vi "FileFunctions.AddDateToFile.vi"   [LabVIEW 2016]
types:
  T1 = enum16{"open", "replace", "create", "open or create", "replace or create", "replace or create with confirmation"}
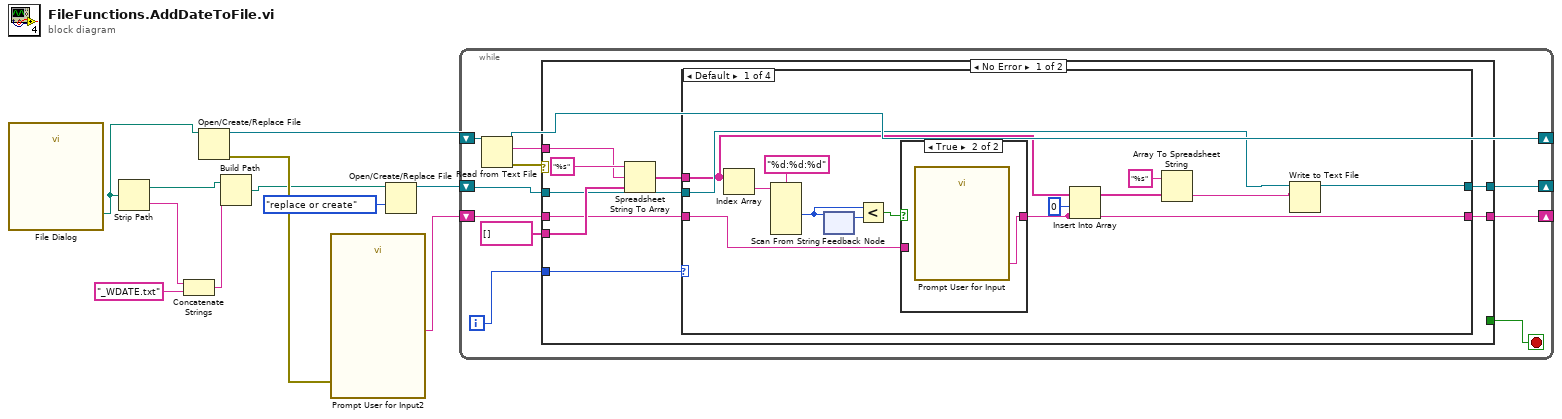
[diagram p0: block diagram]
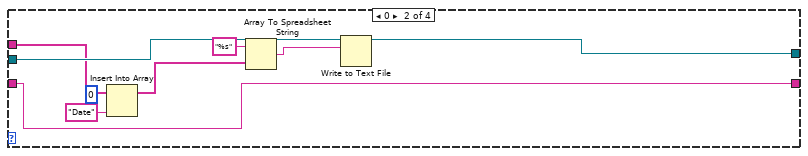
[diagram p3: hidden frame]
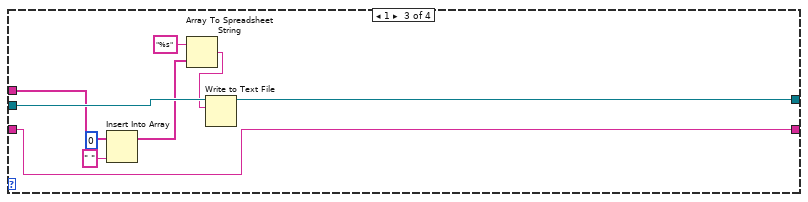
[diagram p4: hidden frame]
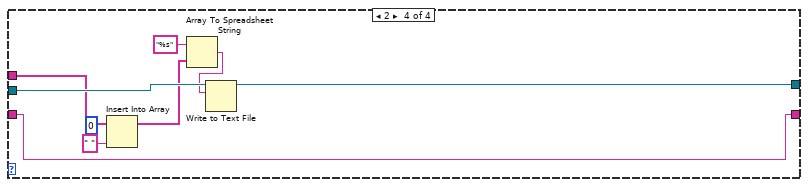
[diagram p5: hidden frame]
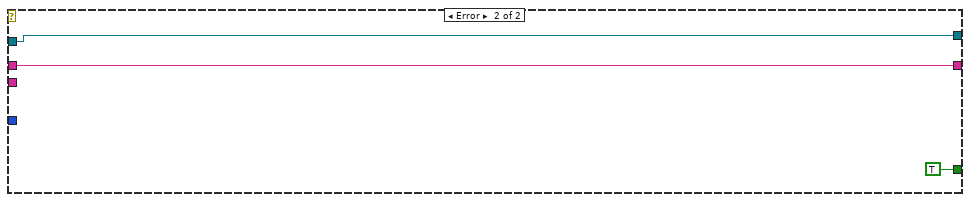
[diagram p6: hidden frame]
diagram:
  n1 = call "File Dialog"() -> ("selected path"=w6:path)  [unwired: 12 in, 3 out]
  n2 = Strip Path(path=w6) -> (stripped path=w5:path, name=w4:string)
  n3 = Concatenate Strings(w4, "_WDATE.txt" ("string")) -> (w3:string)
  n4 = Open/Create/Replace File(file path (use dialog)=w6) -> (refnum out=w7:refnum<file>, error out=w9:errorcluster)  [unwired: 5 in, 1 out]
  n5 = Build Path(base path=w5, name or relative path=w3) -> (appended path=w1:path)
  n6 = call "Prompt User for Input2"("error in (no error)"=w9) -> ("Date"=w8:string)  [unwired: 16 in, 2 out]
  n7 = Open/Create/Replace File(file path (use dialog)=w1, operation (0:open)=T1."replace or create") -> (refnum out=w11:refnum<file>)  [unwired: 4 in, 2 out]
  n8 = while {
    shift-right: [w21] -> _
    shift-left: w7 -> [w20]
    shift-right: [w19] -> _
    shift-left: w11 -> [w18]
    shift-right: [w15] -> _
    shift-left: w8 -> [w14]
    i -> [w16]
    stop <- w12 stop-if-true
    n9 = Read from Text File(file (use dialog)=w20) -> (refnum out=w21:refnum<file>, text=w17:string, error out=w13:errorcluster)  [unwired: 3 in, 1 out]
    n10 = case shown="No Error" w13 {
      tunnel: string[] [] ("format string") -> [w31 _]
      tunnel: [w29 w75] -> w19
      tunnel: w18 -> [w28 w75]
      tunnel: w17 -> [w27 _]
      tunnel: w16 -> [w26 _]
      tunnel: [w24 w76] -> w15
      tunnel: w14 -> [w23 w76]
      tunnel: [_ TRUE] -> w12
      frame No Error {
        n11 = Spreadsheet String To Array(format string="%s", spreadsheet string=w27, array type (2D Dbl)=w31) -> (array=w25:string[])  [unwired: 1 in]
        n12 = case shown="Default" w26 {
          tunnel: [w38 w56 w65 w74] -> w29
          tunnel: w28 -> [w39 w55 w64 w73]
          tunnel: w25 -> [w36 w54 w63 w72]
          tunnel: [w33 w52 w61 w70] -> w24
          tunnel: w23 -> [w40 w52 w61 w70]
          frame Default {
            n13 = Index Array(array=w36) -> (element=w45:string)  [unwired: 1 in]
            n14 = Scan From String(format string="%d:%d:%d", input string=w45) -> (output 1=w43:i32)  [unwired: 7 in, 3 out]
            n15 = feedback-in #1(w43) -> ()
            n16 = feedback #1() -> (w42:i32)  [unwired: 1 in]
            n17 = Less?(x=w43, y=w42) -> (x < y?=w41:bool)
            n18 = case shown="True" w41 {
              tunnel: [w46 w47] -> w33
              tunnel: w40 -> [w46 _]
              frame False {
              }
              frame True {
                n19 = call "Prompt User for Input"() -> ("Date"=w47:string)  [unwired: 17 in, 2 out]
              }
            }
            n20 = Insert Into Array(array=w36, index=0, new element=w33) -> (w34:string[])
            n21 = Array To Spreadsheet String(array=w34, 3:"%s" ("format string")) -> (spreadsheet string=w37:string)  [unwired: 1 in]
            n22 = Write to Text File(file (use dialog)=w39, text=w37) -> (refnum out=w38:refnum<file>)  [unwired: 2 in, 2 out]
          }
          frame 0 {
            n23 = Insert Into Array(array=w54, index=0, new element="Date" ("new element/subarray")) -> (w50:string[])
            n24 = Array To Spreadsheet String(array=w50, 3:"%s" ("format string")) -> (spreadsheet string=w49:string)  [unwired: 1 in]
            n25 = Write to Text File(file (use dialog)=w55, text=w49) -> (refnum out=w56:refnum<file>)  [unwired: 2 in, 2 out]
          }
          frame 1 {
            n26 = Insert Into Array(array=w63, index=0, new element=" " ("new element/subarray")) -> (w59:string[])
            n27 = Array To Spreadsheet String(array=w59, 3:"%s" ("format string")) -> (spreadsheet string=w58:string)  [unwired: 1 in]
            n28 = Write to Text File(file (use dialog)=w64, text=w58) -> (refnum out=w65:refnum<file>)  [unwired: 2 in, 2 out]
          }
          frame 2 {
            n29 = Insert Into Array(array=w72, index=0, new element=" " ("new element/subarray")) -> (w67:string[])
            n30 = Array To Spreadsheet String(array=w67, 3:"%s" ("format string")) -> (spreadsheet string=w68:string)  [unwired: 1 in]
            n31 = Write to Text File(file (use dialog)=w73, text=w68) -> (refnum out=w74:refnum<file>)  [unwired: 2 in, 2 out]
          }
        }
      }
      frame Error {
      }
    }
  }
